vi "Prezentacja_OnDemand_.vi"() -> ()   [LabVIEW 2015]
uses:
  <vilib>/Instr/_visa.llb/VISA Configure Serial Port (Instr).vi
  <vilib>/Analysis/NI_AALBase.lvlib
panel:
  in  "stop":bool
  in  "Tab Control":enum32{"Main", "Service"}(tab)
  in  "oversampling":u16(ring) items=["1", "4", "256", "2048"]
  in  "gain":u16(ring) items=["1", "2", "16", "64"]
  out "mean":dbl format="%.6f"
  out "standard deviation":dbl=nan format="%.6f"
  out "Measurement":dbl(graph)
  out "error out":errorcluster={"status"=TRUE, "code"=-1073807343, "source"="VISA Open in 2_OnDemand_Diff.vi"}
  in  "VISA resource name":refnum<visa-resource-name>="COM7"
  out "answer":string
  in  "Clear":bool
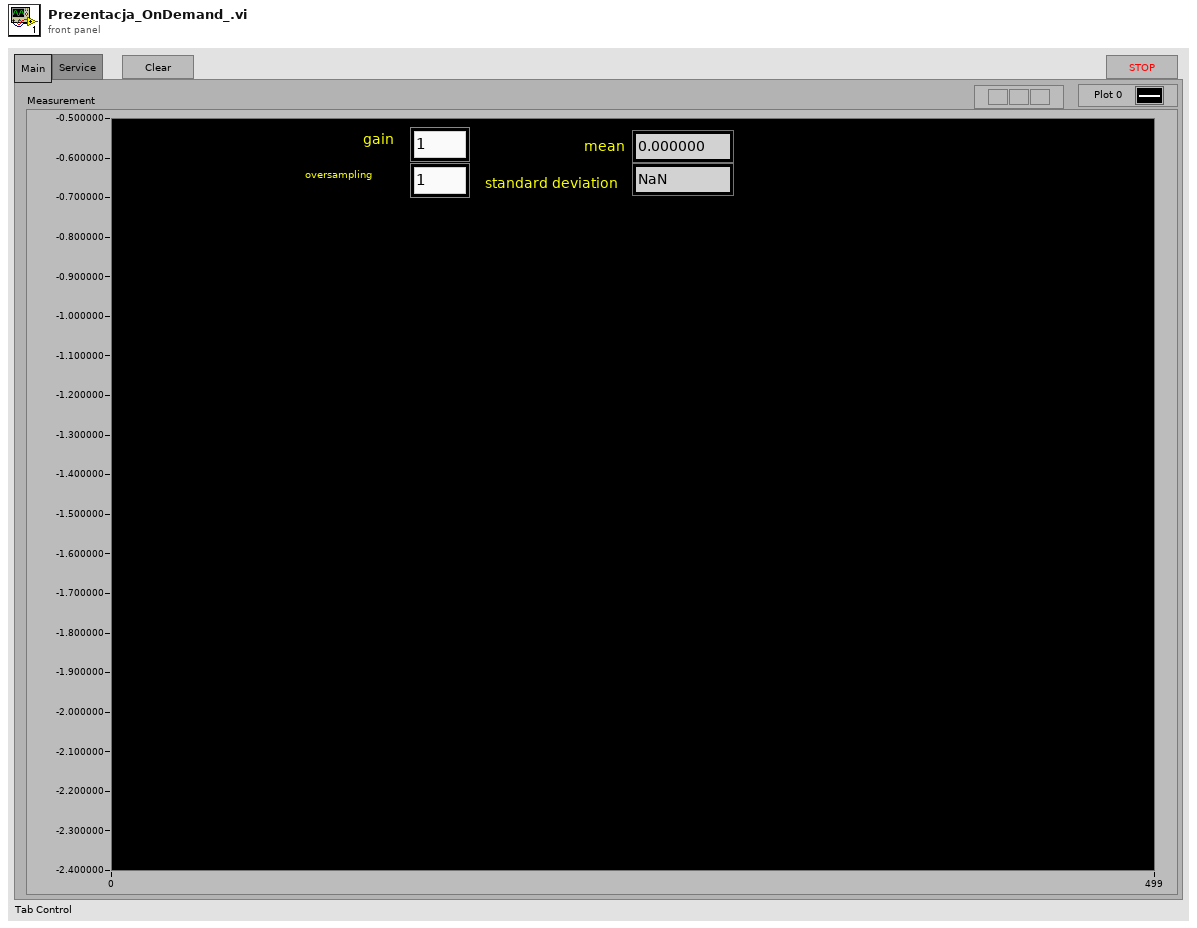
[diagram p1: front panel]
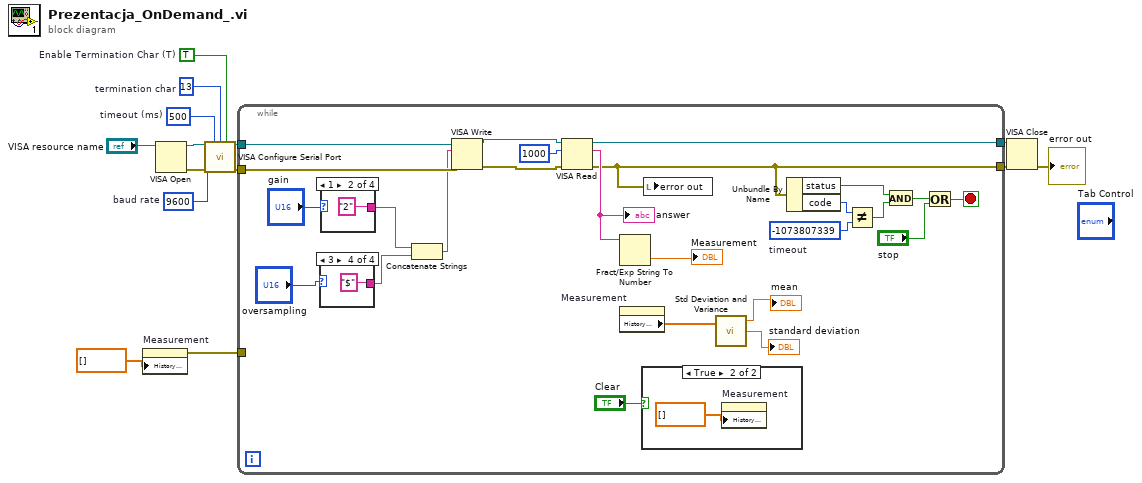
[diagram p0: block diagram]
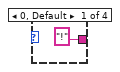
[diagram p2: hidden frame]
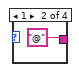
[diagram p3: hidden frame]
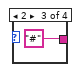
[diagram p4: hidden frame]
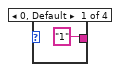
[diagram p5: hidden frame]
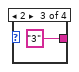
[diagram p6: hidden frame]
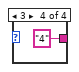
[diagram p7: hidden frame]
diagram:
  w3 = u32 9600  # baud rate
  w4 = u32 500  # timeout (ms)
  w10 = TRUE  # Enable Termination Char (T)
  w11 = u8 13  # termination char
  n1 = property on="Measurement" class="WFChart (strict)"("History Data"=dbl[] []) -> (error out=w1:errorcluster)  [unwired: 2 in, 1 out]
  n2 = VISA Open(VISA resource name="VISA resource name") -> (VISA resource name=w13:refnum<visa-resource-name>, error out=w14:errorcluster)  [unwired: 4 in]
  n3 = call-poly "VISA Configure Serial Port"("VISA resource name"=w13, "timeout (10sec)"=w4, "termination char\n(0xA = '\\n' = LF)"=w11, "Enable Termination\nChar (T)"=w10, "baud rate (9600)"=w3, "error in (no error)"=w14) -> ("VISA resource name out"=w7:refnum<visa-resource-name>, "error out"=w6:errorcluster)  [unwired: 8 in]
  n4 = while {
    tunnel: w7 -> [w38]
    tunnel: [w39] -> w9
    tunnel: w6 -> [w37]
    tunnel: [w28] -> w8
    tunnel: w1 -> [_]
    stop <- w22 stop-if-true
    w26 = -1073807339  # timeout
    n5 = case shown="3" "oversampling" {
      tunnel: ["!" ("write buffer") "@" ("write buffer") "#" ("write buffer") "$" ("write buffer")] -> w15
      frame 0, Default {
      }
      frame 1 {
      }
      frame 2 {
      }
      frame 3 {
      }
    }
    n6 = case shown="1" "gain" {
      tunnel: ["1" ("write buffer") "2" ("write buffer") "3" ("write buffer") "4" ("write buffer")] -> w16
      frame 0, Default {
      }
      frame 1 {
      }
      frame 2 {
      }
      frame 3 {
      }
    }
    n7 = Concatenate Strings(w16, w15) -> (w17:string)
    n8 = VISA Write(VISA resource name=w38, write buffer=w17, error in (no error)=w37) -> (VISA resource name out=w34:refnum<visa-resource-name>, error out=w33:errorcluster)  [unwired: 1 out]
    n9 = VISA Read(VISA resource name=w34, byte count=u32 1000, error in (no error)=w33) -> (VISA resource name out=w39:refnum<visa-resource-name>, read buffer=w35:string, error out=w28:errorcluster)  [unwired: 1 out]
    "answer" <- w35
    n10 = Fract/Exp String To Number(string=w35) -> (number=→"Measurement":dbl)  [unwired: 3 in, 1 out]
    n11 = property on="Measurement" class="WFChart (strict)"() -> ("History Data"=w32:dbl[])  [unwired: 2 in, 2 out]
    n12 = case shown="True" "Clear" {
      frame False {
      }
      frame True {
        n13 = property on="Measurement" class="WFChart (strict)"("History Data"=dbl[] []) -> ()  [unwired: 2 in, 2 out]
      }
    }
    n14 = local write "error out"(w28) -> ()
    n15 = call <vilib>:"Std Deviation and Variance.vi"("X"=w32) -> ("mean"=→"mean":dbl, "standard deviation"=→"standard deviation":dbl)  [unwired: 1 in, 1 out]
    n16 = Unbundle By Name(w28) -> ("status"=w24:bool, "code"=w27:i32)
    n17 = Not Equal?(x=w27, y=w26) -> (x != y?=w25:bool)
    n18 = And(x=w24, y=w25) -> (x .and. y?=w23:bool)
    n19 = Or(x=w23, y="stop") -> (x .or. y?=w22:bool)
  }
  n20 = VISA Close(VISA resource name=w9, error in (no error)=w8) -> (error out=→"error out":errorcluster)
